vi "JogOverLeftRight.vi"(11 "Numeric":dbl) -> ()   [LabVIEW 2020]
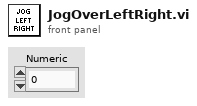
[diagram p1: front panel]
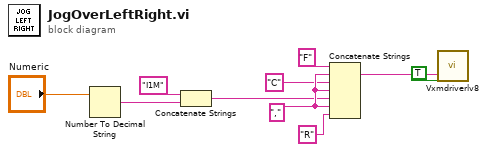
[diagram p0: block diagram]
diagram:
  w9 = ","
  n1 = Number To Decimal String(number="Numeric") -> (decimal integer string=w6:string)  [unwired: 1 in]
  n2 = Concatenate Strings("I1M" ("string"), w6) -> (w7:string)
  n3 = Concatenate Strings("F", w9, "C", w9, w7, w9, "R" ("string")) -> (w4:string)
  n4 = call "Vxmdriverlv8.Vi"("Send\nchars\nto port"=TRUE, "Chars to send"=w4) -> ()  [unwired: 20 in, 6 out]
